vi "LED_randwait.vi"(6 "FPGA I/O In":refnum<k21>="IO Module\\D0 0", 8 "seed":u32=4294967295, 9 "Testpulse Time Delay (20 ns ticks)":u32=15, 10 "Testpulse duration (20 ns ticks)":u32=1, 11 "Testpulser On/Off":bool) -> (0 "Total number of pulses sent":u64, 7 "Is Test Pulse?":bool)   [LabVIEW 2012]
uses:
  <vilib>/rvi/eio/common/nirviEmuTemplateMethod_errors.vi
  <vilib>/eio/EIONode/EIONode.xnode
panel:
  in  "reset":bool
  out "Testpulse Separation (20 ns ticks)":u32=500
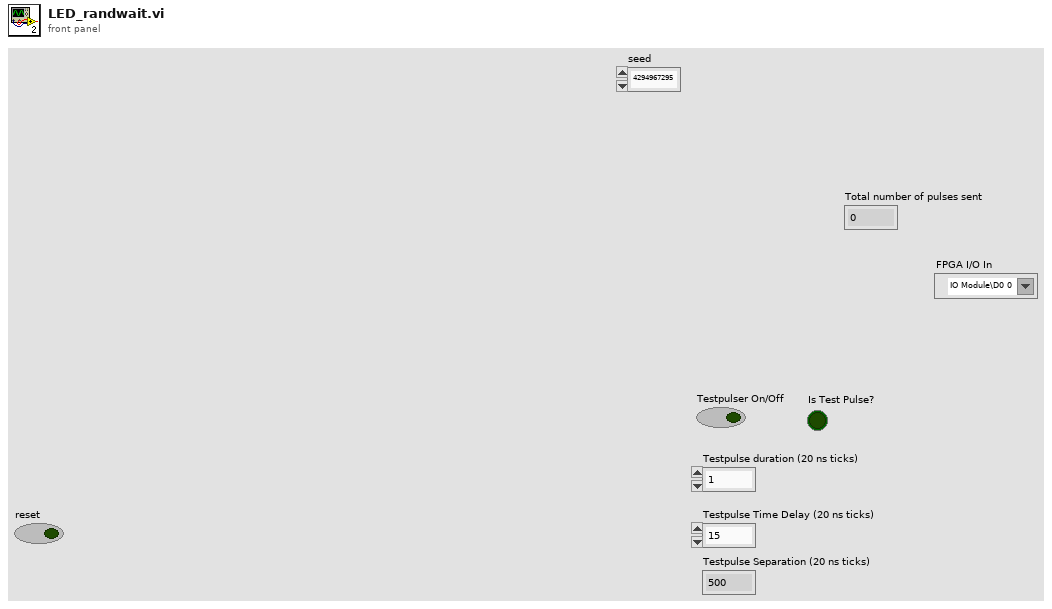
[diagram p1: front panel]
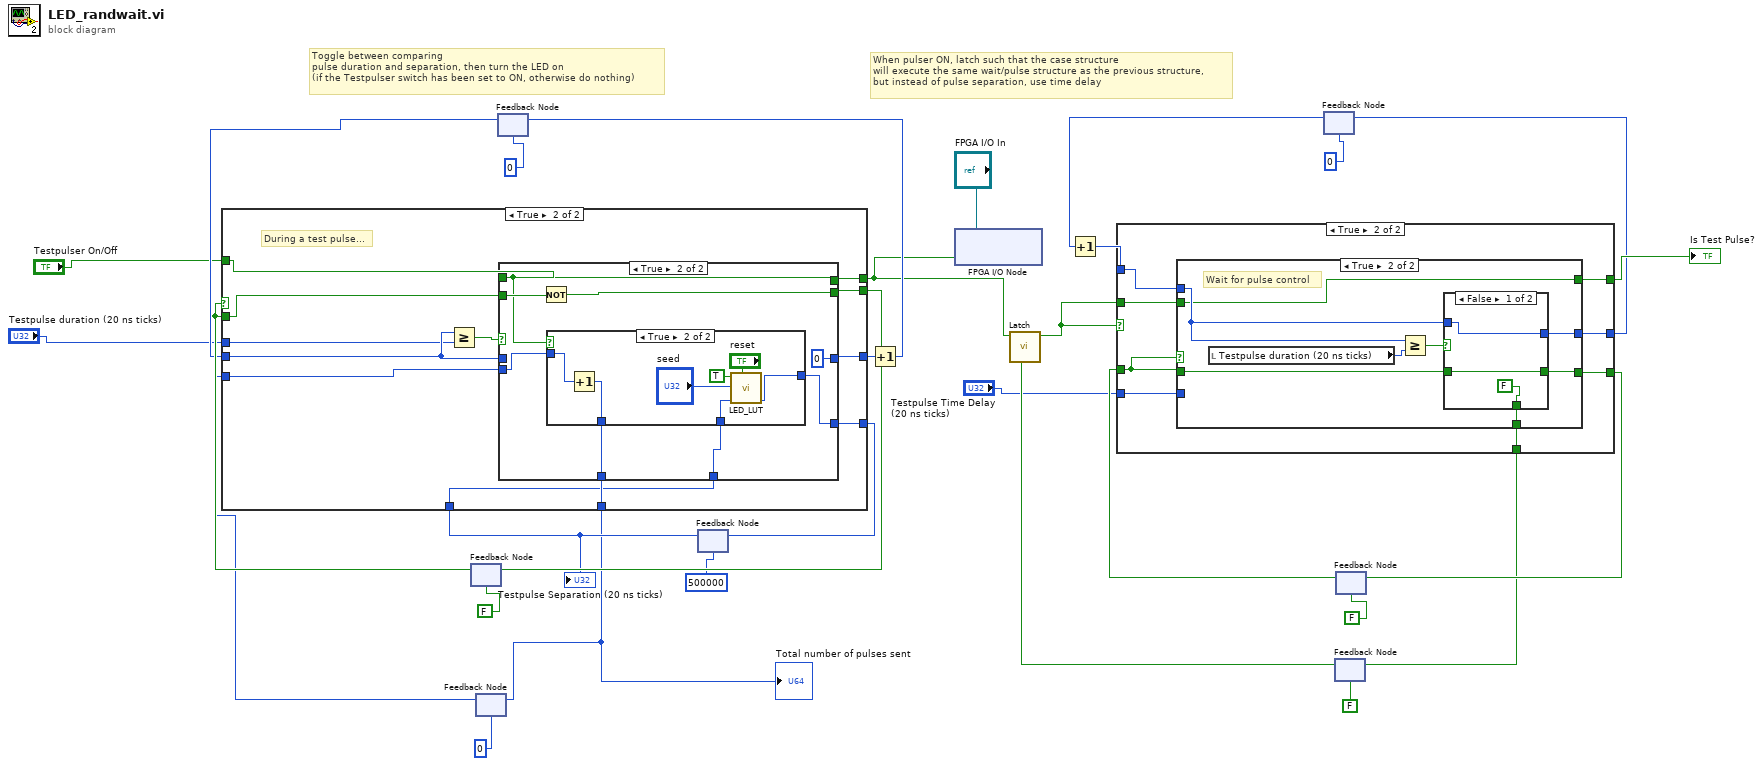
[diagram p0: block diagram]
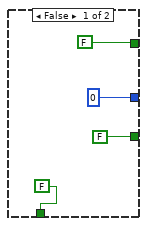
[diagram p2: hidden frame]
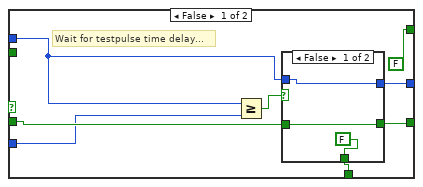
[diagram p3: hidden frame]
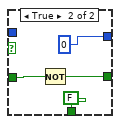
[diagram p4: hidden frame]
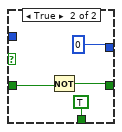
[diagram p5: hidden frame]
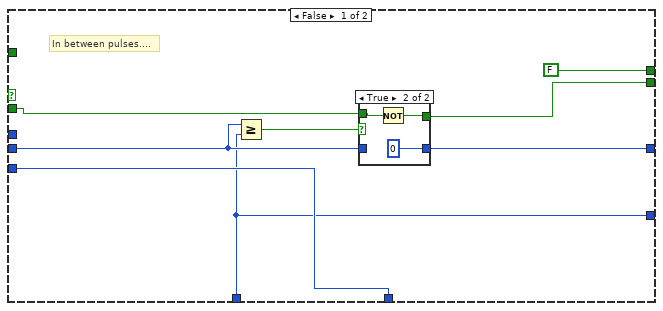
[diagram p6: hidden frame]
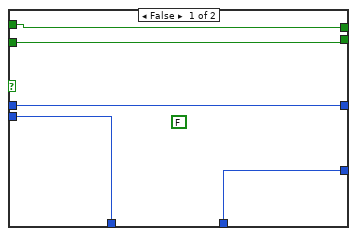
[diagram p8: hidden frame]
diagram:
  # "Toggle between comparing \npulse duration and separation, then turn the LED on\n(if the Testpulser switch has been set to ON, otherwise do nothing)"
  # "When pulser ON, latch such that the case structure\nwill execute the same wait/pulse structure as the previous structure, \nbut instead of pulse separation, use time delay"
  n1 = feedback #1(FALSE) -> (w27:bool)
  n2 = feedback #2(u64 0) -> (w2:u64)
  n3 = feedback #3(u32 0) -> (w14:u32)
  n4 = feedback #4(u32 500000 ("Randomly generated testpulse separation out")) -> (w4:u32)
  "Testpulse Separation (20 ns ticks)" <- w4
  n5 = case shown="True" w27 {
    tunnel: w14 -> [w35 w53]
    tunnel: [w38 w54] -> w12
    tunnel: [w37 w55] -> w19
    tunnel: [FALSE ("IO Module\\D0 0") w48] -> w10
    tunnel: w27 -> [w33 w51]
    tunnel: w2 -> [w32 w50]
    tunnel: [w32 w49] -> w3
    tunnel: [w31 w47] -> w9
    tunnel: w4 -> [w31 w46]
    tunnel: "Testpulser On/Off" -> [_ w45]
    tunnel: "Testpulse duration (20 ns ticks)" -> [_ w44]
    frame False {
      # "In between pulses...."
      n6 = Greater Or Equal?(x=w35, y=w31) -> (x >= y?=w34:bool)
      n7 = case shown="True" w34 {
        tunnel: [w40 u32 0] -> w38
        tunnel: w35 -> [w40 _]
        tunnel: [w39 w42] -> w37
        tunnel: w33 -> [w39 w41]
        frame False {
        }
        frame True {
          n8 = Not(x=w41) -> (.not. x?=w42:bool)
        }
      }
    }
    frame True {
      # "During a test pulse..."
      n9 = Greater Or Equal?(x=w53, y=w44) -> (x >= y?=w52:bool)
      n10 = case shown="True" w52 {
        tunnel: w53 -> [w60 _]
        tunnel: [w59 w68] -> w55
        tunnel: [w60 u32 0] -> w54
        tunnel: w51 -> [w59 w66]
        tunnel: w50 -> [w58 w65]
        tunnel: [w58 w64] -> w49
        tunnel: w45 -> [w57 w63]
        tunnel: [w57 w63] -> w48
        tunnel: [w56 w62] -> w47
        tunnel: w46 -> [w56 w61]
        frame False {
          (unwired) FALSE
        }
        frame True {
          n11 = Not(x=w66) -> (.not. x?=w68:bool)
          n12 = case shown="True" w63 {
            tunnel: w65 -> [w70 w77]
            tunnel: [w70 w76] -> w64
            tunnel: [w69 w73] -> w62
            tunnel: w61 -> [w69 w72]
            frame False {
            }
            frame True {
              n13 = Increment(x=w77) -> (x+1=w76:u64)
              n14 = call "LED_LUT.vi"("reset"="reset", "Previous value of randomly generated testpulse separation"=w72, "seed"="seed", "Need a new random number?"=TRUE) -> ("Randomly generated testpulse separation out"=w73:u32)  [unwired: 7 in]
            }
          }
        }
      }
    }
  }
  "Total number of pulses sent" <- w3
  n15 = feedback-in #1(w19) -> ()
  n16 = feedback-in #2(w3) -> ()
  n17 = feedback-in #4(w9) -> ()
  n18 = Increment(x=w12) -> (x+1=w13:u32)
  n19 = feedback-in #3(w13) -> ()
  n20 = xnode "FPGA I/O Node"("I/O Item"=w10, "FPGA I/O In"="FPGA I/O In") -> ()  [unwired: 1 out]
  n21 = feedback #5(u32 0) -> (w25:u32)
  n22 = Increment(x=w25) -> (x+1=w24:u32)
  n23 = feedback #6(FALSE) -> (w16:bool)
  n24 = call "Latch.vi"("Reset"=w16, "Input"=w10) -> ("Output"=w15:bool)  [unwired: 9 in]
  n25 = feedback #7(FALSE) -> (w21:bool)
  n26 = case shown="True" w15 {
    tunnel: w15 -> [_ w84]
    tunnel: [FALSE w86] -> w30
    tunnel: w24 -> [_ w87]
    tunnel: [u32 0 w85] -> w23
    tunnel: w21 -> [_ w89]
    tunnel: [FALSE w88] -> w20
    tunnel: [FALSE w83] -> w17
    tunnel: "Testpulse Time Delay (20 ns ticks)" -> [_ w82]
    frame False {
    }
    frame True {
      n27 = case shown="True" w89 {
        tunnel: w89 -> [w96 w109]
        tunnel: [w95 w108] -> w88
        tunnel: w87 -> [w92 w110]
        tunnel: [FALSE w106] -> w86
        tunnel: [w93 w107] -> w85
        tunnel: w84 -> [_ w106]
        tunnel: [w91 w105] -> w83
        tunnel: w82 -> [w90 _]
        frame False {
          # "Wait for testpulse time delay..."
          n28 = Greater Or Equal?(x=w92, y=w90) -> (x >= y?=w97:bool)
          n29 = case shown="False" w97 {
            tunnel: w96 -> [w100 w104]
            tunnel: [w100 w103] -> w95
            tunnel: [w99 u32 0] -> w93
            tunnel: w92 -> [w99 _]
            tunnel: [FALSE FALSE] -> w91
            frame False {
            }
            frame True {
              n30 = Not(x=w104) -> (.not. x?=w103:bool)
            }
          }
        }
        frame True {
          # "Wait for pulse control"
          n31 = local read "Testpulse duration (20 ns ticks)"() -> (w112:u32)
          n32 = Greater Or Equal?(x=w110, y=w112) -> (x >= y?=w111:bool)
          n33 = case shown="False" w111 {
            tunnel: w110 -> [w114 _]
            tunnel: w109 -> [w115 w118]
            tunnel: [w115 w117] -> w108
            tunnel: [w114 u32 0] -> w107
            tunnel: [FALSE TRUE] -> w105
            frame False {
            }
            frame True {
              n34 = Not(x=w118) -> (.not. x?=w117:bool)
            }
          }
        }
      }
    }
  }
  "Is Test Pulse?" <- w30
  n35 = feedback-in #5(w23) -> ()
  n36 = feedback-in #6(w17) -> ()
  n37 = feedback-in #7(w20) -> ()
